vi "Read Wiring Configuration.vi"(8 "error in (no error)":errorcluster, 11 "Control Experiment in":refnum<class "Control Experiment.lvclass">) -> (0 "error out":errorcluster, 2 "Wiring Configuration":T1, 3 "Control Experiment out":refnum<class "Control Experiment.lvclass">)   [LabVIEW 2016, in "Control Experiment.lvclass"]
uses:
  Control Experiment.lvclass
  Typedefs/Wiring Description--cluster.ctl
  Control Experiment.lvclass/Control Experiment.ctl
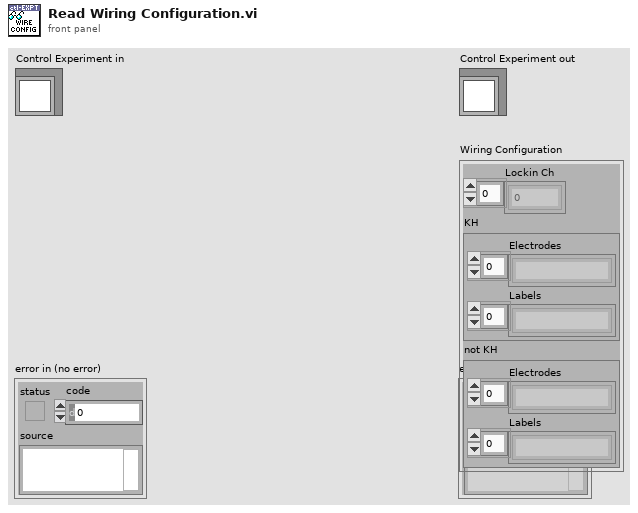
[diagram p1: front panel]
types:
  T1 = typedef "Control Experiment.lvclass/Wiring Description--cluster.ctl" = cluster{"Lockin Ch":i32[], "KH":cluster{"Electrodes":string[], "Labels":string[]}, "not KH":cluster{"Electrodes":string[], "Labels":string[]}}
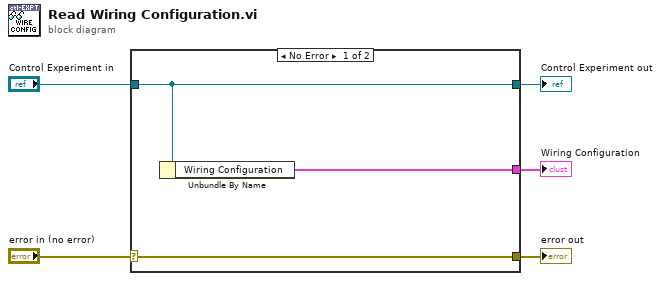
[diagram p0: block diagram]
diagram:
  n1 = case shown="No Error" "error in (no error)" {
    selector: "error in (no error)" -> [w8 w9]
    tunnel: [w8 w9] -> w4
    tunnel: [w7 w10] -> w2
    tunnel: "Control Experiment in" -> [w7 w10]
    tunnel: [w6 _] -> w1
    frame No Error {
      n2 = Unbundle By Name(w7) -> ("Wiring Configuration"=w6:T1)
    }
    frame Error {
    }
  }
  "error out" <- w4
  "Control Experiment out" <- w2
  "Wiring Configuration" <- w1
